vi "Main.vi"() -> ()   [LabVIEW 2012]
uses:
  MeasureDialogButton.ctl
  SourceDialogButton.ctl
  TriggerDialogButton.ctl
  DUTDisplayData.ctl
  DUTDialogButton.ctl
  LogDialogButton.ctl
  driver/Public/Controls/SMU.ctl
  DisplayDataGlobalAction.ctl
  UIActionQueueElement.ctl
  UIAction.ctl
  SetupGlobalAction.ctl
  HardwareActionQueueElement.ctl
  HardwareAction.ctl
  HardwareAbortGlobalAction.ctl
  LogActionQueueElement.ctl
  LogAction.ctl
  DisplayDataChartDialogGlobalAction.ctl
  driver/Keithley-2602.lvlib
  libs/LV-Utilities/LV-Utilities.lvlib
panel:
  in  "CREATE CHART":bool
  in  "Hardware START":bool
  out "Hardware Running?":bool
  in  "LOG START":bool
  out "Log Running?":bool
  out "Digital IO Port":bool[](array[boolean])
  out "Setup File":path
  in  "RESET":bool
  in  "SAVE":bool
  in  "OPEN":bool
  in  "SHOW LOG DIALOG":T1
  in  "SHOW DUT DIALOG":T2
  in  "SHOW SOURCE DIALOG":T3
  in  "SHOW TRIGGER DIALOG":T4
  in  "SHOW MEASURE DIALOG":T5
  out "System SMU B DUT Display Data":T6[](array[typedef]) {"Resistance (Ohm)" format="%_4p"; "Current (A)" format="%_4p"; "Voltage (V)" format="%_4p"}
  out "System SMU A DUT Display Data":T6[](array[typedef]) {"Resistance (Ohm)" format="%_4p"; "Current (A)" format="%_4p"; "Voltage (V)" format="%_4p"}
  out "Log File":path
  in  "DONE":bool
  # "RUN"
  # "LOG"
  # "DIGITAL IO"
  # "1"
  # "2"
  # "3"
  # "4"
  # "5"
  # "6"
  # "7"
  # "8"
  # "9"
  # "10"
  # "11"
  # "12"
  # "13"
  # "14"
  # "SETUP"
  # "SMU B"
  # "SMU A"
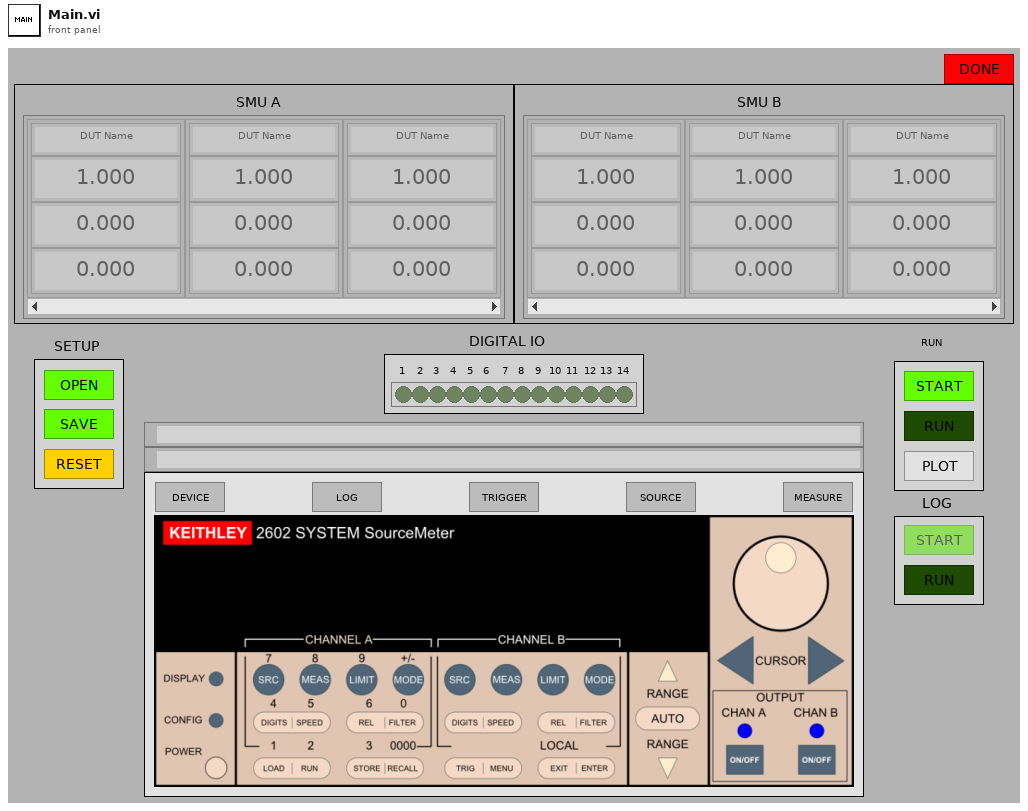
[diagram p1: front panel]
types:
  T1 = typedef "LogDialogButton.ctl" = bool
  T2 = typedef "DUTDialogButton.ctl" = bool
  T3 = typedef "SourceDialogButton.ctl" = bool
  T4 = typedef "TriggerDialogButton.ctl" = bool
  T5 = typedef "MeasureDialogButton.ctl" = bool
  T6 = typedef "DUTDisplayData.ctl" = cluster{"Name":string, "Voltage (V)":dbl, "Current (A)":dbl, "Resistance (Ohm)":dbl}
  T7 = typedef "ExecutableConfiguration.ctl" = cluster{"GPIB ID":u8, "GPIB Board":u8, "Default Data Folder":path, "Default Setup Folder":path}
  T8 = typedef "DataStructures.ctl" = cluster{"Display Data":refnum<notifier>, "Log Data":refnum<queue>}
  T9 = typedef "ActionQueues.ctl" = cluster{"UI Action":refnum<queue>, "Hardware Action":refnum<queue>, "Log Action":refnum<queue>}
  T10 = typedef "DisplayDataGlobalAction.ctl" = enum16{"Get", "Set"}
  T11 = typedef "Keithley-2602.lvlib/SMU.ctl" = enum16{"A", "B"}
  T12 = typedef "SetupGlobalAction.ctl" = enum16{"Get", "Set", "Reset"}
  T13 = enum8{"Enabled", "Disabled", "Disabled and Grayed Out"}
  T14 = typedef "UIActionQueueElement.ctl" = cluster{"Action":T15, "Data":variant}
  T15 = typedef "UIAction.ctl" = enum16{"Initialize", "Configure Trigger", "Configure Measure", "Configure Source", "Configure DUT", "Configure Log", "Configure Open", "Configure Save", "Configure Reset", "Hardware Start", "Hardware Started", "Hardware Stop", "Hardware Stopped", "Log Arm", "Log Start", "Log Started", "Log Stop", "Log Stopped", "Create Chart", "Error", "Shutdown"}
  T16 = typedef "HardwareActionQueueElement.ctl" = cluster{"Action":T17, "Data":variant}
  T17 = typedef "HardwareAction.ctl" = enum16{"Initialize", "Start", "Run", "Stop", "Error", "Shutdown"}
  T18 = typedef "HardwareAbortGlobalAction.ctl" = enum16{"Set", "Get"}
  T19 = typedef "LogActionQueueElement.ctl" = cluster{"Action":T20, "Data":variant}
  T20 = typedef "LogAction.ctl" = enum16{"Initialize", "Start", "Arm", "Create", "Write", "Close", "Rearm", "Stop", "Error", "Shutdown"}
  T21 = typedef "DisplayDataChartDialogGlobalAction.ctl" = enum16{"Create", "Close"}
  T22 = typedef "HardwareDisplayData.ctl" = cluster{"DUT Names":string[][], "SMU":dbl[][], "Port":bool[]}
  T23 = typedef "Setup.ctl" = cluster{"DUT":T24, "Log":T26, "Trigger":T34, "Sources":T40[], "Measures":T42[]}
  T24 = typedef "DUTConfiguration.ctl" = cluster{"Count":u32, "Wirings":T25[], "Names":string[][]}
  T25 = typedef "Keithley-2602.lvlib/SMUSense.ctl" = enum16{"Local (2-wire)", "Remote (4-wire)", "Calibration"}
  T26 = typedef "LogConfiguration.ctl" = cluster{"Start":T27, "Rollover":T30, "Stop":T32}
  T27 = typedef "LogStartConfiguration.ctl" = cluster{"Trigger Type":T28, "Timer (sec)":dbl, "Digital IO Line":u8, "Digital IO Edge":T29}
  T28 = typedef "LogStartTriggerType.ctl" = enum16{"Immediate", "User", "Timer", "Digital IO"}
  T29 = typedef "LogDigitalIOTriggerEdge.ctl" = enum16{"Rising", "Falling"}
  T30 = typedef "LogRolloverConfiguration.ctl" = cluster{"Trigger Type":T31, "Timer (sec)":dbl, "File Size (MB)":u32, "Digital IO Line":u8, "Digital IO Edge":T29}
  T31 = typedef "LogRolloverTriggerType.ctl" = enum16{"None", "Timer", "File Size", "Digital IO"}
  T32 = typedef "LogStopConfiguration.ctl" = cluster{"Trigger Type":T33, "Timer (sec)":dbl, "File Size (MB)":u32, "Digital IO Line":u8, "Digital IO Edge":T29}
  T33 = typedef "LogStopTriggerType.ctl" = enum16{"None", "User", "Timer", "File Size", "Digital IO"}
  T34 = typedef "TriggerConfiguration.ctl" = cluster{"Input":T35, "Output":T38}
  T35 = typedef "TriggerInputConfiguration.ctl" = cluster{"Type":T36, "Timeout (ms)":u32, "Delay (ms)":u32, "Digital IO Line (1-14)":u8, "Digital IO Mode":T37}
  T36 = typedef "TriggerInputType.ctl" = enum16{"None", "Digital IO", "Bus"}
  T37 = typedef "Keithley-2602.lvlib/TriggerMode.ctl" = enum16{"Falling", "Rising", "Either", "Synchronous"}
  T38 = typedef "TriggerOutputConfiguration.ctl" = cluster{"Type":T39, "Delay (ms)":u32, "Digital IO Line (1-14)":u8, "Digital IO Mode":T37, "Digital IO Pulse Width (sec)":dbl}
  T39 = typedef "TriggerOutputType.ctl" = enum16{"None", "Digital IO", "Bus"}
  T40 = typedef "SourceConfiguration.ctl" = cluster{"Enabled?":bool, "Function":T41, "Level (V or A)":dbl, "Autorange Enabled?":bool, "High Limit (V or A)":dbl, "Low Limit (V or A)":dbl}
  T41 = typedef "SourceFunction.ctl" = enum16{"Voltage", "Current"}
  T42 = typedef "MeasureConfiguration.ctl" = cluster{"Enabled?":bool, "Count":u8, "Interval (sec)":dbl, "Voltage Auto Range Enabled?":bool, "Voltage High Limit (V or A)":dbl, "Voltage Low Limit (V or A)":dbl, "Current Auto Range Enabled?":bool, "Current High Limit (V or A)":dbl, "Current Low Limit (V or A)":dbl}
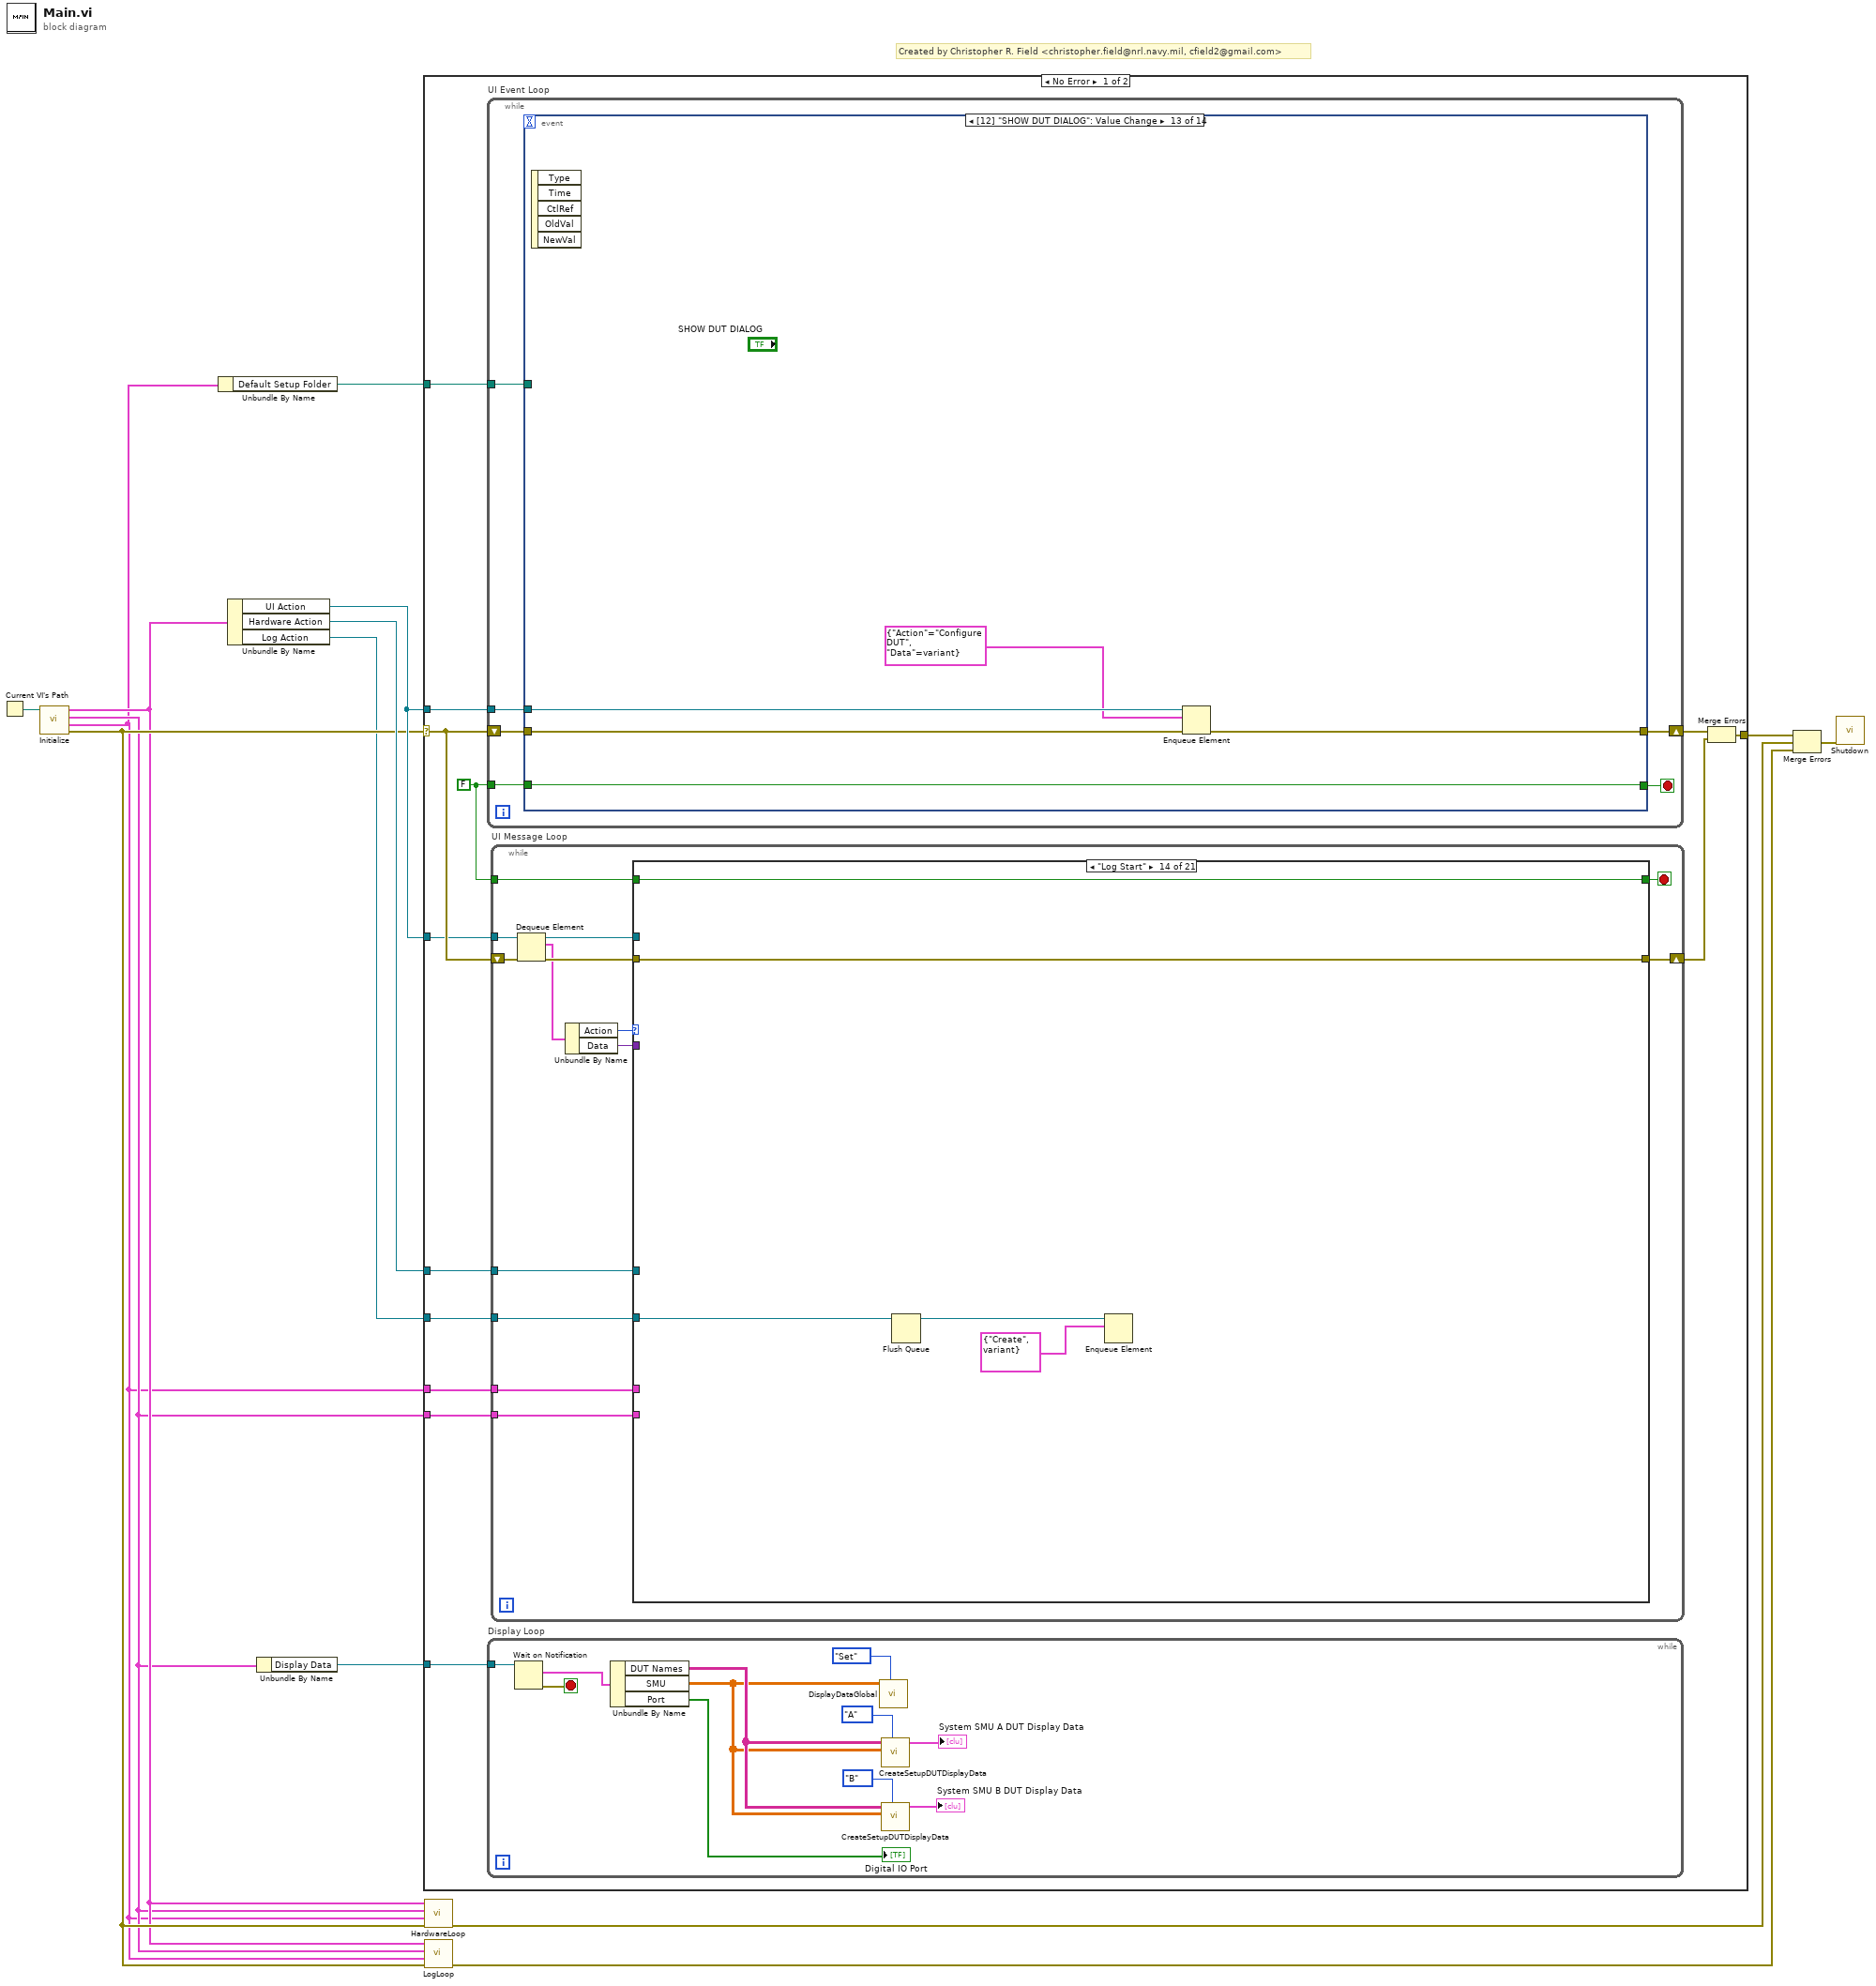
[diagram p0: block diagram]
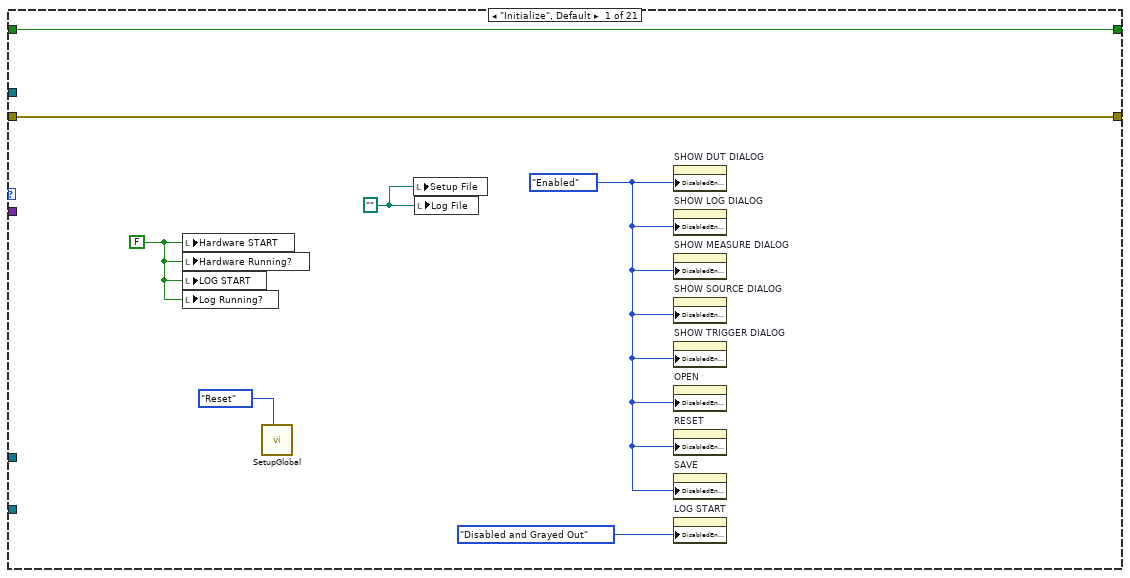
[diagram p2: hidden frame]
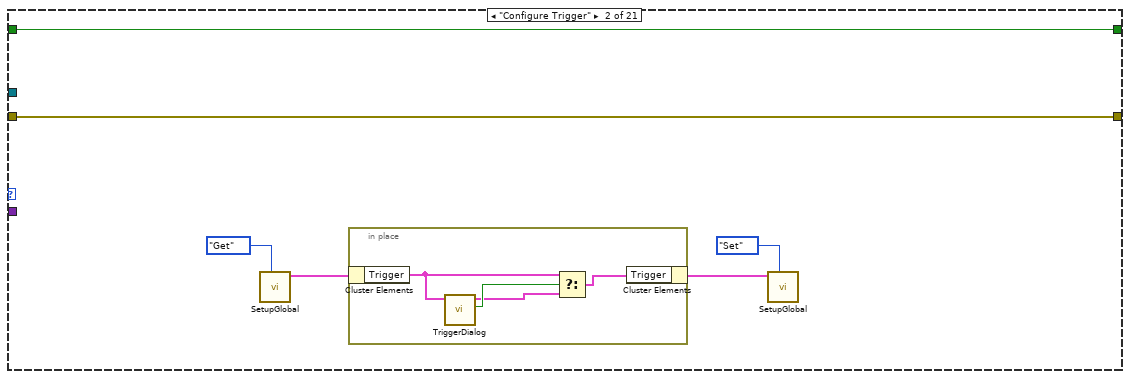
[diagram p3: hidden frame]
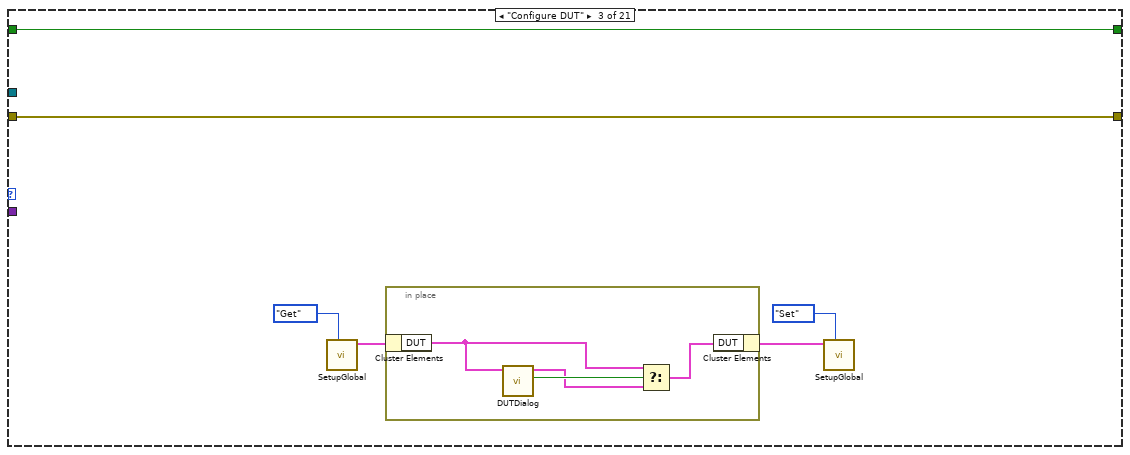
[diagram p4: hidden frame]
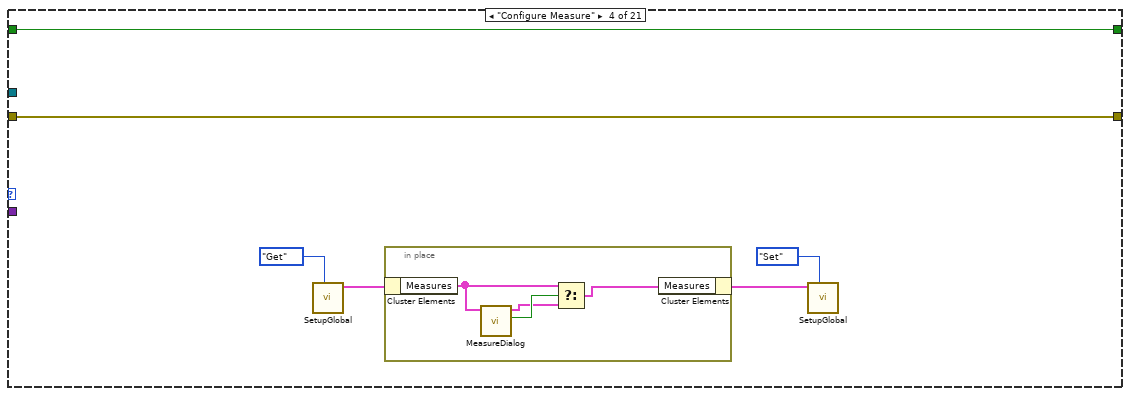
[diagram p5: hidden frame]
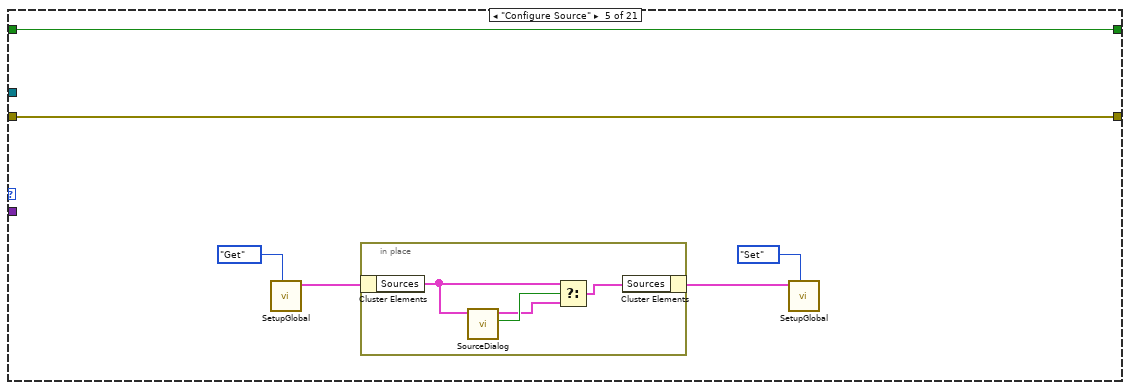
[diagram p6: hidden frame]
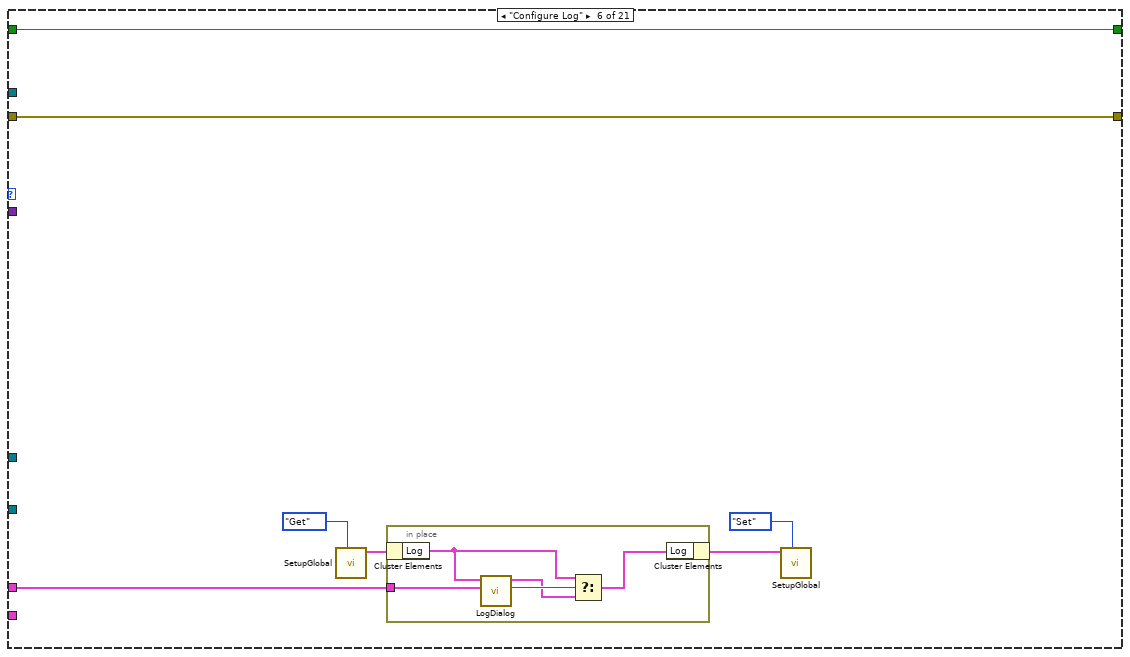
[diagram p7: hidden frame]
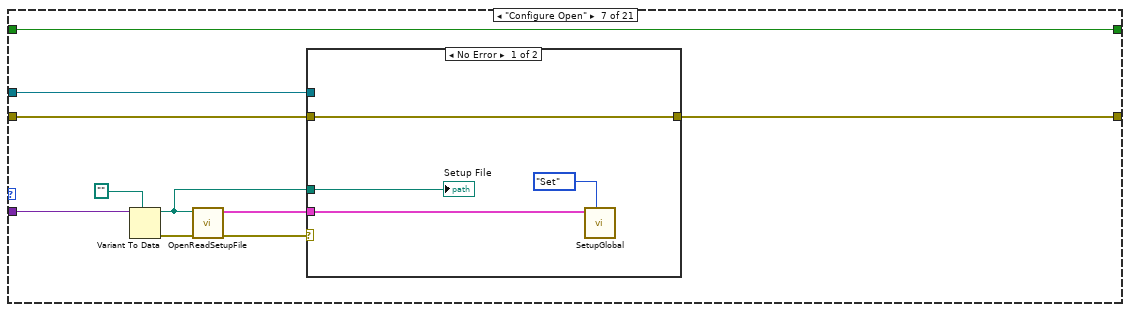
[diagram p8: hidden frame]
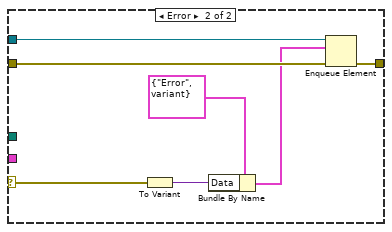
[diagram p9: hidden frame]
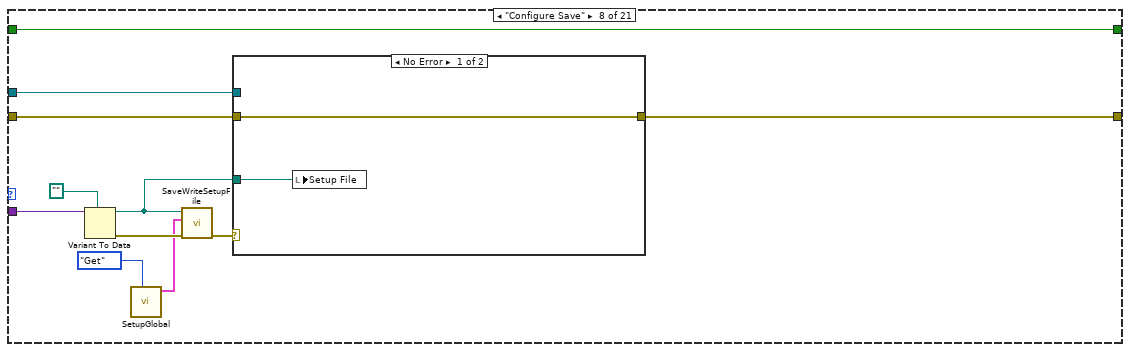
[diagram p10: hidden frame]
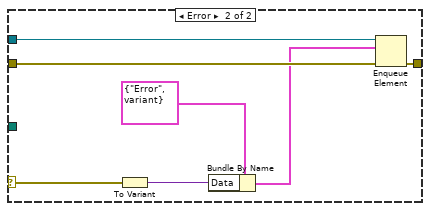
[diagram p11: hidden frame]
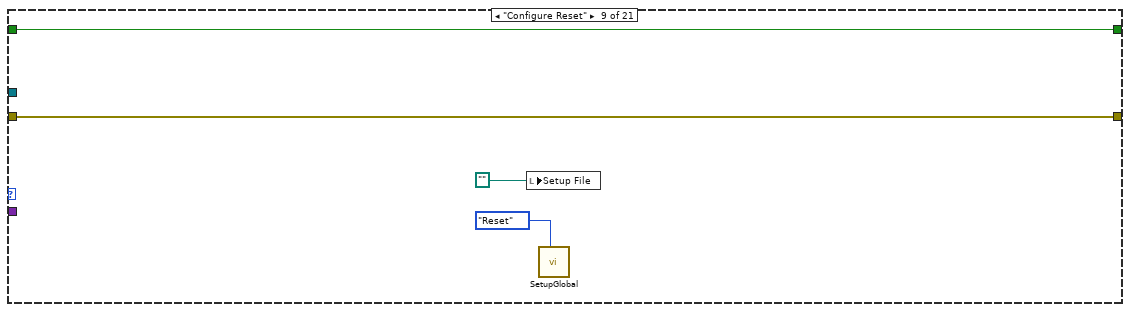
[diagram p12: hidden frame]
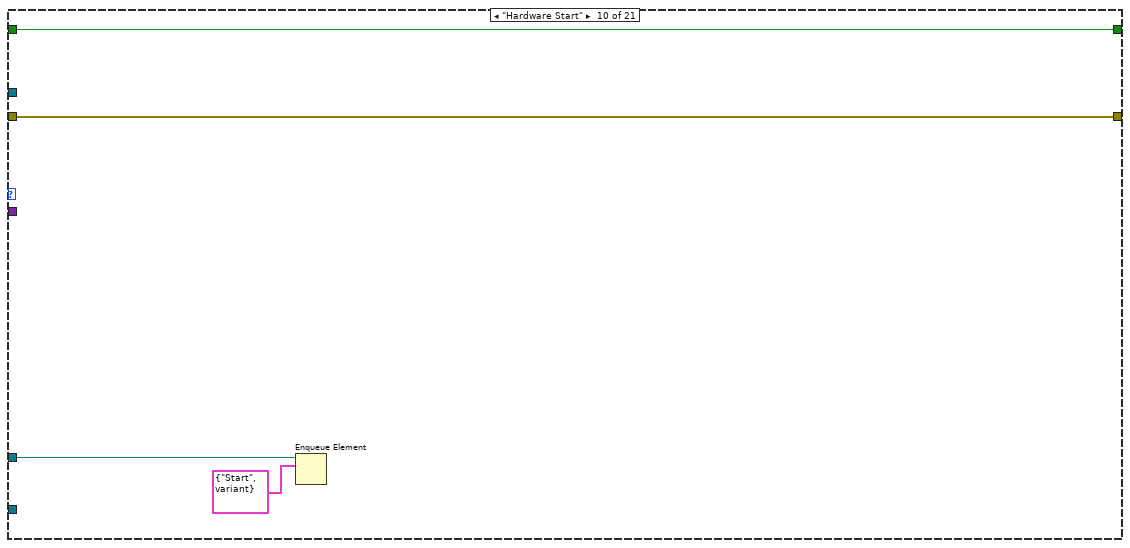
[diagram p13: hidden frame]
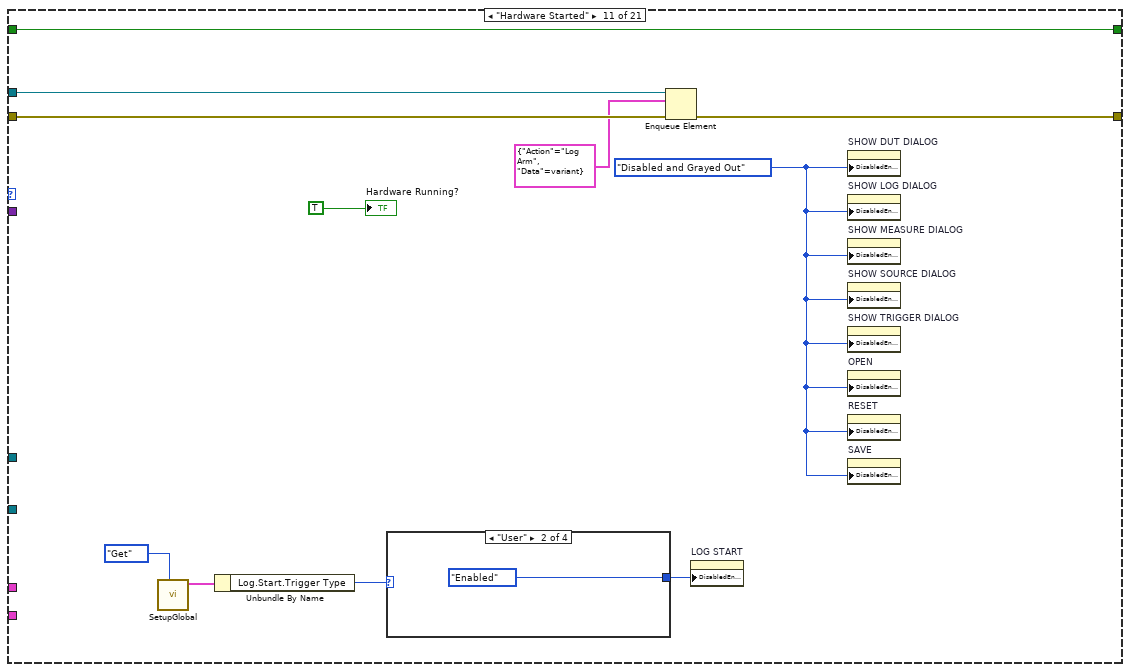
[diagram p14: hidden frame]
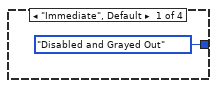
[diagram p15: hidden frame]
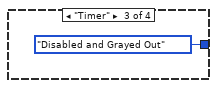
[diagram p16: hidden frame]
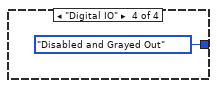
[diagram p17: hidden frame]
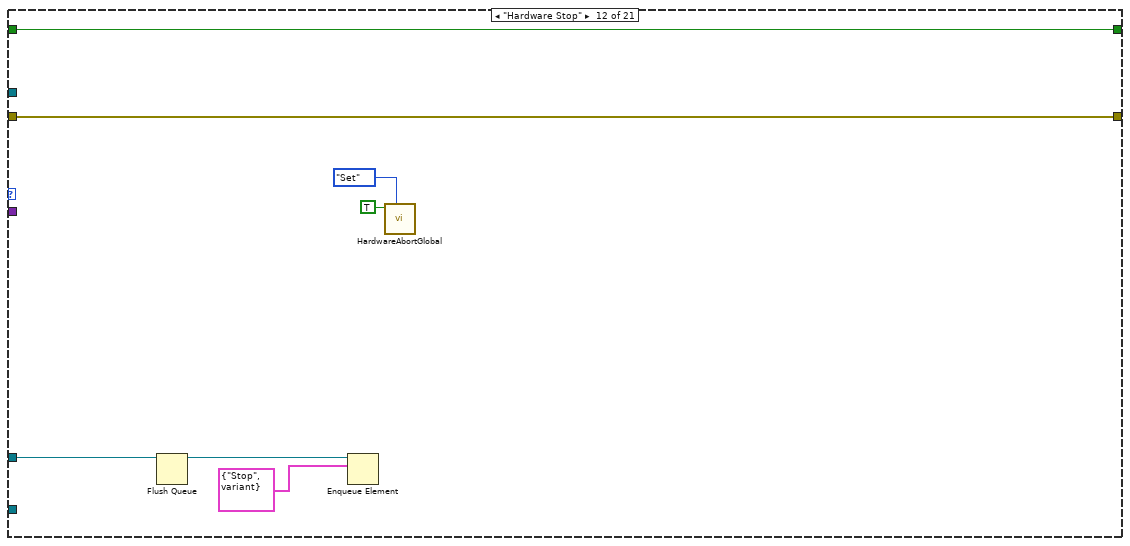
[diagram p18: hidden frame]
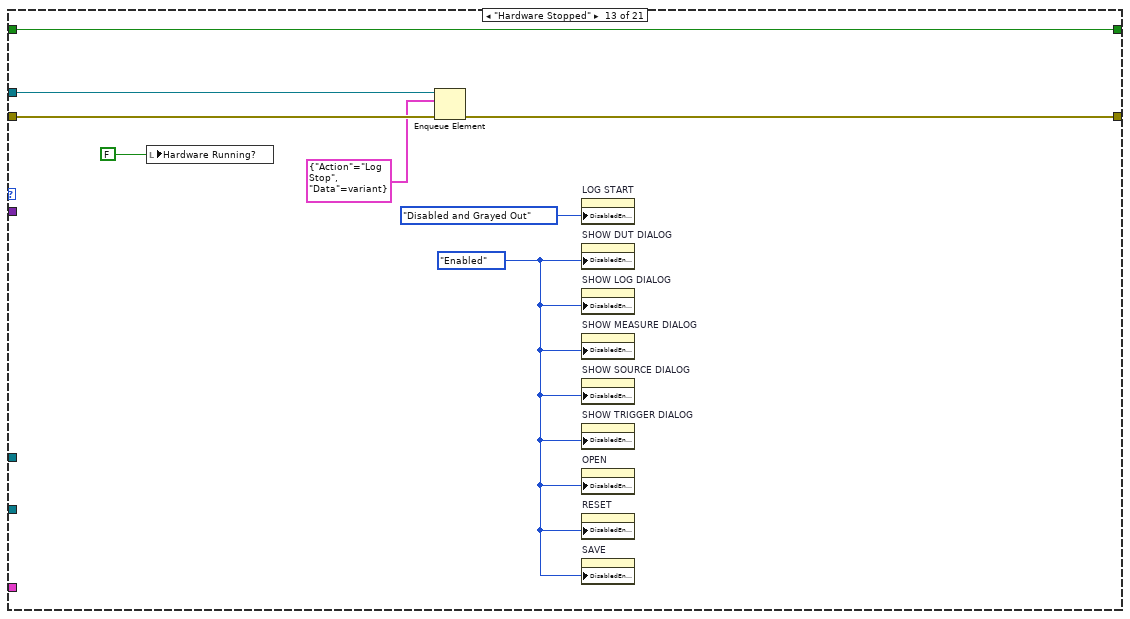
[diagram p19: hidden frame]
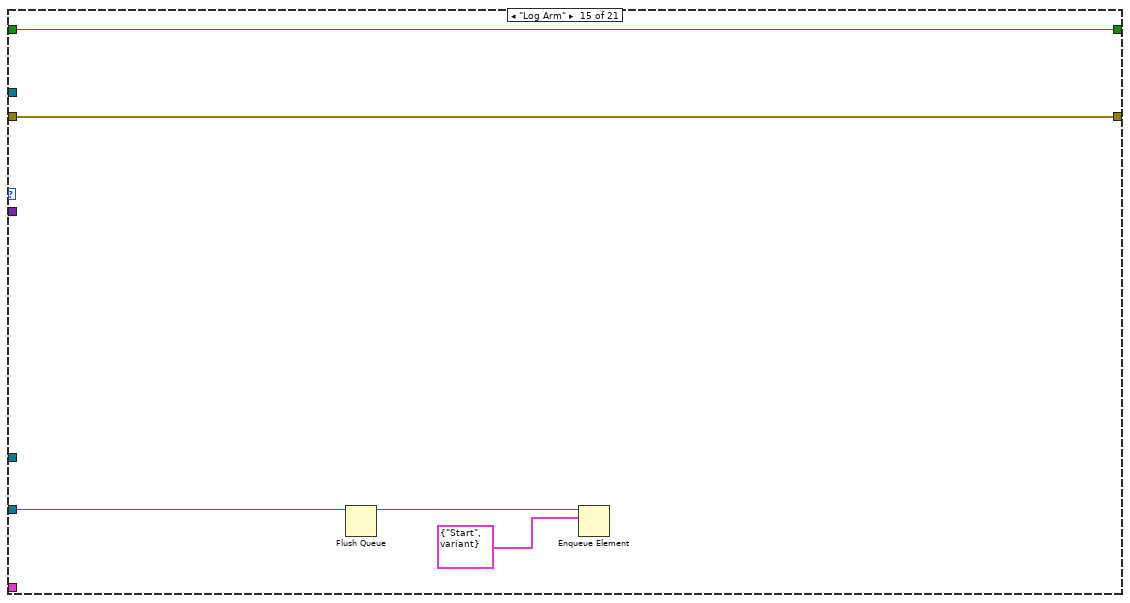
[diagram p20: hidden frame]
diagram:
  # "Created by Christopher R. Field <christopher.field@nrl.navy.mil, cfield2@gmail.com>"
  n1 = Current VI's Path() -> (path=w9:path)
  n2 = call "Initialize.vi"("VI Path"=w9) -> ("Error Out"=w7:errorcluster, "Executable Configuration"=w2:T7, "Data Structures"=w5:T8, "Action Queues"=w6:T9)  [unwired: 7 in]
  n3 = Unbundle By Name(w2) -> ("Default Setup Folder"=w1:path)
  n4 = Unbundle By Name(w6) -> ("UI Action"=w14:refnum<queue>, "Hardware Action"=w10:refnum<queue>, "Log Action"=w3:refnum<queue>)
  n5 = Unbundle By Name(w5) -> ("Display Data"=w8:refnum<notifier>)
  n6 = case shown="No Error" w7 {
    selector: w7 -> [w25 w373]
    tunnel: [w26 w373] -> w13
    tunnel: w14 -> [w22 _]
    tunnel: w14 -> [w21 _]
    tunnel: w10 -> [w20 _]
    tunnel: w8 -> [w19 _]
    tunnel: w5 -> [w18 _]
    tunnel: w2 -> [w17 _]
    tunnel: w3 -> [w16 _]
    tunnel: w1 -> [w15 _]
    frame No Error {
      w23 = FALSE
      n7 = while "UI Event Loop" {
        tunnel: w23 -> [w267]
        shift-right: [w264] -> w27
        shift-left: w25 -> [w265]
        tunnel: w21 -> [w263]
        tunnel: w15 -> [w262]
        stop <- w266 stop-if-true
        n8 = event shown="[12] \"SHOW DUT DIALOG\": Value Change" {
          selector: _ -> [_ _ _ _ _ _ _ _ _ _ _ _ _ _]
          dyn-events: _ -> [_ _ _ _ _ _ _ _ _ _ _ _ _ _]
          timeout: _ -> [_ _ _ _ _ _ _ _ _ _ _ _ _ _]
          tunnel: w267 -> [w269 w275 w280 w294 w310 w326 w331 w336 w338 w352 w357 w359 w367 w369]
          tunnel: [w269 w274 w280 w294 w310 w326 w331 w336 w338 w351 w357 w359 w367 w369] -> w266
          tunnel: w265 -> [w268 w271 w282 w285 w312 w324 w329 w334 w340 w347 w355 w361 w365 w371]
          tunnel: [w268 w272 w281 w286 w311 w323 w328 w333 w339 w350 w354 w360 w364 w370] -> w264
          tunnel: w263 -> [_ w273 w283 w287 w313 w325 w330 w335 w341 w348 w356 w362 w366 w372]
          tunnel: w262 -> [_ _ _ w284 w303 _ _ _ _ _ _ _ _ _]
          event Timeout {
            n9 = event-data() -> ()  [unwired: 1 in, 2 out]
          }
          event Panel Close? {
            n10 = event-data() -> ()  [unwired: 1 in, 3 out]
            n11 = Not(x=w275) -> (.not. x?=w274:bool)
            n12 = Enqueue Element(queue=w273, element=T14 {"Action"=enum."Shutdown", "Data"=variant}, error in (no error)=w271) -> (error out=w272:errorcluster)  [unwired: 1 in, 2 out]
            n13 = event-data("Discard?"=w274) -> ()  [unwired: 1 in, 1 out]
          }
          event "LOG START": Value Change {
            n14 = event-data() -> ()  [unwired: 1 in, 5 out]
            n15 = Select(t=T14 {"Action"=enum."Log Start", "Data"=variant} ("element"), s="LOG START", f=T14 {"Action"=enum."Log Stop", "Data"=variant} ("element")) -> (s? t:f=w276:T14)
            n16 = Enqueue Element(queue=w283, element=w276, error in (no error)=w282) -> (error out=w281:errorcluster)  [unwired: 1 in, 2 out]
          }
          event "OPEN": Value Change {
            n17 = event-data() -> ()  [unwired: 1 in, 5 out]
            n18 = call "SelectFile.vi"("Button Label"="Open", "Prompt"="Select Setup File", "File Description"="Setup File", "File Extension (.*)"=".xml", "Start Path"=w284) -> ("Cancelled?"=w289:bool, "Selected File Path"=w288:path)  [unwired: 4 in, 1 out]
            n19 = case shown="False" w289 {
              tunnel: w287 -> [w301 _]
              tunnel: w285 -> [w300 w302]
              tunnel: [w299 w302] -> w286
              tunnel: w288 -> [w296 _]
              frame False {
                n20 = To Variant(anything=w296) -> (Variant=w297:variant)
                n21 = Bundle By Name(cluster=T14 {"Action"=enum."Configure Open", "Data"=variant} ("element"), "Data"=w297) -> (w295:T14)
                n22 = Enqueue Element(queue=w301, element=w295, error in (no error)=w300) -> (error out=w299:errorcluster)  [unwired: 1 in, 2 out]
              }
              frame True {
              }
            }
          }
          event "SAVE": Value Change {
            n23 = event-data() -> ()  [unwired: 1 in, 5 out]
            n24 = call "SelectFile.vi"("Button Label"="Save", "Prompt"="Select Setup File", "File Description"="Setup File", "File Extension (.*)"=".xml", "Start Path"=w303) -> ("Cancelled?"=w305:bool, "Selected File Path"=w304:path)  [unwired: 4 in, 1 out]
            n25 = case shown="False" w305 {
              tunnel: w313 -> [w320 _]
              tunnel: w312 -> [w319 w321]
              tunnel: [w318 w321] -> w311
              tunnel: w304 -> [w315 _]
              frame False {
                n26 = To Variant(anything=w315) -> (Variant=w316:variant)
                n27 = Bundle By Name(cluster=T14 {"Action"=enum."Configure Save", "Data"=variant} ("element"), "Data"=w316) -> (w314:T14)
                n28 = Enqueue Element(queue=w320, element=w314, error in (no error)=w319) -> (error out=w318:errorcluster)  [unwired: 1 in, 2 out]
              }
              frame True {
              }
            }
          }
          event "RESET": Value Change {
            n29 = event-data() -> ()  [unwired: 1 in, 5 out]
            n30 = Enqueue Element(queue=w325, element=T14 {"Action"=enum."Configure Reset", "Data"=variant}, error in (no error)=w324) -> (error out=w323:errorcluster)  [unwired: 1 in, 2 out]
          }
          event Value Change {
            n31 = event-data() -> ()  [unwired: 1 in, 1 out]
            n32 = Enqueue Element(queue=w330, element=T14 {"Action"=enum."Configure Measure", "Data"=variant}, error in (no error)=w329) -> (error out=w328:errorcluster)  [unwired: 1 in, 2 out]
          }
          event Value Change {
            n33 = event-data() -> ()  [unwired: 1 in, 5 out]
            n34 = Enqueue Element(queue=w335, element=T14 {"Action"=enum."Configure Source", "Data"=variant}, error in (no error)=w334) -> (error out=w333:errorcluster)  [unwired: 1 in, 2 out]
          }
          event "Hardware START": Value Change {
            n35 = event-data() -> ()  [unwired: 1 in, 1 out]
            n36 = Select(t=T14 {"Action"=enum."Hardware Start", "Data"=variant} ("UI Action Queue Element"), s="Hardware START", f=T14 {"Action"=enum."Hardware Stop", "Data"=variant} ("UI Action Queue Element")) -> (s? t:f=w337:T14)
            n37 = Enqueue Element(queue=w341, element=w337, error in (no error)=w340) -> (error out=w339:errorcluster)  [unwired: 1 in, 2 out]
          }
          event "DONE": Value Change {
            n38 = event-data() -> ()  [unwired: 1 in, 5 out]
            n39 = Not(x=w352) -> (.not. x?=w351:bool)
            n40 = Flush Queue(queue=w348, error in (no error)=w347) -> (queue out=w345:refnum<queue>, error out=w346:errorcluster)  [unwired: 1 out]
            n41 = Enqueue Element(queue=w345, element=T14 {"Action"=enum."Shutdown", "Data"=variant}, error in (no error)=w346) -> (error out=w350:errorcluster)  [unwired: 1 in, 2 out]
          }
          event Value Change {
            n42 = event-data() -> ()  [unwired: 1 in, 5 out]
            n43 = Enqueue Element(queue=w356, element=T14 {"Action"=enum."Configure Trigger", "Data"=variant}, error in (no error)=w355) -> (error out=w354:errorcluster)  [unwired: 1 in, 2 out]
          }
          event "CREATE CHART": Value Change {
            n44 = event-data() -> ()  [unwired: 1 in, 5 out]
            n45 = Enqueue Element(queue=w362, element=T14 {"Action"=enum."Create Chart", "Data"=variant} ("UI Action Queue Element"), error in (no error)=w361) -> (error out=w360:errorcluster)  [unwired: 1 in, 2 out]
          }
          event Value Change {
            n46 = event-data() -> ()  [unwired: 1 in, 5 out]
            n47 = Enqueue Element(queue=w366, element=T14 {"Action"=enum."Configure DUT", "Data"=variant}, error in (no error)=w365) -> (error out=w364:errorcluster)  [unwired: 1 in, 2 out]
          }
          event Value Change {
            n48 = event-data() -> ()  [unwired: 1 in, 5 out]
            n49 = Enqueue Element(queue=w372, element=T14 {"Action"=enum."Configure Log", "Data"=variant}, error in (no error)=w371) -> (error out=w370:errorcluster)  [unwired: 1 in, 2 out]
          }
        }
      }
      n50 = while "Display Loop" {
        tunnel: w19 -> [w38]
        stop <- w37 stop-if-true
        n51 = Wait on Notification(notifier=w38) -> (notification=w36:T22, error out=w37:errorcluster)  [unwired: 3 in, 2 out]
        n52 = Unbundle By Name(w36) -> ("DUT Names"=w32:string[][], "SMU"=w29:dbl[][], "Port"=→"Digital IO Port":bool[])
        n53 = call "DisplayDataGlobal.vi"("Action"=DisplayDataGlobalAction."Set", "Set Value"=w29) -> ()  [unwired: 9 in, 1 out]
        n54 = call "CreateSetupDUTDisplayData.vi"("SMU"=SMU."A", "SMU Data"=w29, "DUT Names"=w32) -> ("DUT Display Data"=→"System SMU A DUT Display Data":T6[])  [unwired: 8 in]
        n55 = call "CreateSetupDUTDisplayData.vi"("SMU"=SMU."B", "SMU Data"=w29, "DUT Names"=w32) -> ("DUT Display Data"=→"System SMU B DUT Display Data":T6[])  [unwired: 8 in]
      }
      n56 = while "UI Message Loop" {
        shift-right: [w51] -> w24
        shift-left: w25 -> [w49]
        tunnel: w23 -> [w52]
        tunnel: w22 -> [w48]
        tunnel: w20 -> [w42]
        tunnel: w18 -> [w41]
        tunnel: w17 -> [w40]
        tunnel: w16 -> [w39]
        stop <- w50 stop-if-true
        n57 = Dequeue Element(queue=w48, error in (no error)=w49) -> (queue out=w46:refnum<queue>, element=w45:T14, error out=w47:errorcluster)  [unwired: 1 in, 1 out]
        n58 = Unbundle By Name(w45) -> ("Action"=w44:T15, "Data"=w43:variant)
        n59 = case shown="\"Log Start\"" w44 {
          tunnel: w52 -> [w59 w65 w75 w85 w95 w106 w121 w143 w156 w160 w171 w182 w190 w195 w200 w210 w221 w228 w239 w243 w257]
          tunnel: w47 -> [w58 w64 w74 w84 w94 w105 w113 w136 w155 w159 w167 w181 w187 w194 w197 w209 w220 w229 w238 w241 w254]
          tunnel: [w58 w64 w74 w84 w94 w105 w112 w135 w155 w159 w166 w181 w186 w194 w197 w209 w220 w229 w238 w241 w253] -> w51
          tunnel: [w59 w65 w75 w85 w95 w106 w121 w143 w156 w160 w171 w182 w190 w195 w200 w210 w221 w228 w239 w243 w256] -> w50
          tunnel: w46 -> [_ _ _ _ _ _ w114 w137 _ _ w168 _ w188 _ _ _ _ _ _ _ w255]
          tunnel: w43 -> [_ _ _ _ _ _ w120 w141 _ _ _ _ _ _ _ w208 _ _ _ w242 _]
          tunnel: w42 -> [_ _ _ _ _ _ _ _ _ w158 _ w179 _ _ _ _ _ _ _ _ w252]
          tunnel: w41 -> [_ _ _ _ _ _ _ _ _ _ _ _ _ _ _ _ _ _ _ _ _]
          tunnel: w40 -> [_ _ _ _ _ w104 _ _ _ _ _ _ _ _ _ _ _ _ _ _ _]
          tunnel: w39 -> [_ _ _ _ _ _ _ _ _ _ _ _ _ w193 w198 _ w219 _ _ _ w250]
          frame "Initialize", Default {
            w54 = T13."Enabled" ("Disabled")
            w55 = path ""
            w57 = FALSE ("START")
            n60 = local write "Hardware START"(w57) -> ()
            n61 = local write "Hardware Running?"(w57) -> ()
            n62 = local write "LOG START"(w57) -> ()
            n63 = local write "Log Running?"(w57) -> ()
            n64 = call "SetupGlobal.vi"("Action"=SetupGlobalAction."Reset") -> ()  [unwired: 10 in, 1 out]
            n65 = local write "Setup File"(w55) -> ()
            n66 = local write "Log File"(w55) -> ()
            n67 = property on="SHOW DUT DIALOG" class="Bool"("DisabledEnum"=w54) -> ()  [unwired: 2 in, 2 out]
            n68 = property on="SHOW LOG DIALOG" class="Bool"("DisabledEnum"=w54) -> ()  [unwired: 2 in, 2 out]
            n69 = property on="SHOW MEASURE DIALOG" class="Bool"("DisabledEnum"=w54) -> ()  [unwired: 2 in, 2 out]
            n70 = property on="SHOW SOURCE DIALOG" class="Bool"("DisabledEnum"=w54) -> ()  [unwired: 2 in, 2 out]
            n71 = property on="SHOW TRIGGER DIALOG" class="Bool"("DisabledEnum"=w54) -> ()  [unwired: 2 in, 2 out]
            n72 = property on="OPEN" class="Bool"("DisabledEnum"=w54) -> ()  [unwired: 2 in, 2 out]
            n73 = property on="RESET" class="Bool"("DisabledEnum"=w54) -> ()  [unwired: 2 in, 2 out]
            n74 = property on="SAVE" class="Bool"("DisabledEnum"=w54) -> ()  [unwired: 2 in, 2 out]
            n75 = property on="LOG START" class="Bool (strict)"("DisabledEnum"=T13."Disabled and Grayed Out" ("Disabled")) -> ()  [unwired: 2 in, 2 out]
          }
          frame "Configure Trigger" {
            n76 = call "SetupGlobal.vi"("Action"=SetupGlobalAction."Get") -> ("Value Out"=w62:T23)  [unwired: 10 in]
            n77 = in-place {
              n78 = in-place-cluster #1(w62) -> ("Trigger"=w66:T34)
              n79 = call "TriggerDialog.vi"("Trigger Configuration In"=w66) -> ("Cancelled"=w69:bool, "Trigger Configuration Out"=w68:T34)  [unwired: 8 in, 1 out]
              n80 = Select(t=w66, s=w69, f=w68) -> (s? t:f=w67:T34)
              n81 = in-place-cluster #1("Trigger"=w67) -> (w61:T23)
            }
            n82 = call "SetupGlobal.vi"("Action"=SetupGlobalAction."Set", "Set Value"=w61) -> ()  [unwired: 9 in, 1 out]
          }
          frame "Configure DUT" {
            n83 = call "SetupGlobal.vi"("Action"=SetupGlobalAction."Get") -> ("Value Out"=w72:T23)  [unwired: 10 in]
            n84 = in-place {
              n85 = in-place-cluster #2(w72) -> ("DUT"=w76:T24)
              n86 = call "DUTDialog.vi"("DUT Configuration In"=w76) -> ("Cancelled?"=w79:bool, "DUT Configuration Out"=w78:T24)  [unwired: 8 in, 1 out]
              n87 = Select(t=w76, s=w79, f=w78) -> (s? t:f=w77:T24)
              n88 = in-place-cluster #2("DUT"=w77) -> (w70:T23)
            }
            n89 = call "SetupGlobal.vi"("Action"=SetupGlobalAction."Set", "Set Value"=w70) -> ()  [unwired: 9 in, 1 out]
          }
          frame "Configure Measure" {
            n90 = call "SetupGlobal.vi"("Action"=SetupGlobalAction."Get") -> ("Value Out"=w82:T23)  [unwired: 10 in]
            n91 = in-place {
              n92 = in-place-cluster #3(w82) -> ("Measures"=w86:T42[])
              n93 = call "MeasureDialog.vi"("Measure Configuration In"=w86) -> ("Cancelled?"=w89:bool, "Measure Configuration Out"=w87:T42[])  [unwired: 8 in, 1 out]
              n94 = Select(t=w86, s=w89, f=w87) -> (s? t:f=w88:T42[])
              n95 = in-place-cluster #3("Measures"=w88) -> (w80:T23)
            }
            n96 = call "SetupGlobal.vi"("Action"=SetupGlobalAction."Set", "Set Value"=w80) -> ()  [unwired: 9 in, 1 out]
          }
          frame "Configure Source" {
            n97 = call "SetupGlobal.vi"("Action"=SetupGlobalAction."Get") -> ("Value Out"=w92:T23)  [unwired: 10 in]
            n98 = in-place {
              n99 = in-place-cluster #4(w92) -> ("Sources"=w96:T40[])
              n100 = call "SourceDialog.vi"("Source Configurations In"=w96) -> ("Cancelled?"=w99:bool, "Source Configurations Out"=w98:T40[])  [unwired: 8 in, 1 out]
              n101 = Select(t=w96, s=w99, f=w98) -> (s? t:f=w97:T40[])
              n102 = in-place-cluster #4("Sources"=w97) -> (w90:T23)
            }
            n103 = call "SetupGlobal.vi"("Action"=SetupGlobalAction."Set", "Set Value"=w90) -> ()  [unwired: 9 in, 1 out]
          }
          frame "Configure Log" {
            n104 = call "SetupGlobal.vi"("Action"=SetupGlobalAction."Get") -> ("Value Out"=w102:T23)  [unwired: 10 in]
            n105 = in-place {
              in-place-border: w104 -> [w108]
              n106 = in-place-cluster #5(w102) -> ("Log"=w107:T26)
              n107 = call "LogDialog.vi"("Executable Configuration"=w108, "Log Configuration In"=w107) -> ("Cancelled?"=w111:bool, "Log Configuration Out"=w110:T26)  [unwired: 7 in, 1 out]
              n108 = Select(t=w107, s=w111, f=w110) -> (s? t:f=w109:T26)
              n109 = in-place-cluster #5("Log"=w109) -> (w100:T23)
            }
            n110 = call "SetupGlobal.vi"("Action"=SetupGlobalAction."Set", "Set Value"=w100) -> ()  [unwired: 9 in, 1 out]
          }
          frame "Configure Open" {
            n111 = Variant To Data(type=path "", Variant=w120) -> (data=w115:path, error out=w118:errorcluster)  [unwired: 1 in]
            n112 = call "OpenReadSetupFile.vi"("Error In"=w118, "Setup File"=w115) -> ("Error Out"=w117:errorcluster, "Setup"=w116:T23)  [unwired: 8 in]
            n113 = case shown="No Error" w117 {
              selector: w117 -> [_ w127]
              tunnel: w116 -> [w122 _]
              tunnel: w115 -> [w125 _]
              tunnel: w114 -> [_ w132]
              tunnel: w113 -> [w124 w131]
              tunnel: [w124 w130] -> w112
              frame No Error {
                n114 = call "SetupGlobal.vi"("Action"=SetupGlobalAction."Set", "Set Value"=w122) -> ()  [unwired: 9 in, 1 out]
                "Setup File" <- w125
              }
              frame Error {
                n115 = To Variant(anything=w127) -> (Variant=w128:variant)
                n116 = Bundle By Name(cluster=T14 {"Action"=enum."Error", "Data"=variant} ("element"), "Data"=w128) -> (w126:T14)
                n117 = Enqueue Element(queue=w132, element=w126, error in (no error)=w131) -> (error out=w130:errorcluster)  [unwired: 1 in, 2 out]
              }
            }
          }
          frame "Configure Save" {
            n118 = Variant To Data(type=path "", Variant=w141) -> (data=w139:path, error out=w140:errorcluster)  [unwired: 1 in]
            n119 = call "SetupGlobal.vi"("Action"=SetupGlobalAction."Get") -> ("Value Out"=w133:T23)  [unwired: 10 in]
            n120 = call "SaveWriteSetupFile.vi"("Error In"=w140, "Setup"=w133, "Save File"=w139) -> ("Error Out"=w138:errorcluster)  [unwired: 8 in]
            n121 = case shown="No Error" w138 {
              selector: w138 -> [_ w147]
              tunnel: w139 -> [w145 _]
              tunnel: w137 -> [_ w152]
              tunnel: w136 -> [w144 w151]
              tunnel: [w144 w150] -> w135
              frame No Error {
                n122 = local write "Setup File"(w145) -> ()
              }
              frame Error {
                n123 = To Variant(anything=w147) -> (Variant=w148:variant)
                n124 = Bundle By Name(cluster=T14 {"Action"=enum."Error", "Data"=variant} ("element"), "Data"=w148) -> (w146:T14)
                n125 = Enqueue Element(queue=w152, element=w146, error in (no error)=w151) -> (error out=w150:errorcluster)  [unwired: 1 in, 2 out]
              }
            }
          }
          frame "Configure Reset" {
            n126 = local write "Setup File"(path "") -> ()
            n127 = call "SetupGlobal.vi"("Action"=SetupGlobalAction."Reset") -> ()  [unwired: 10 in, 1 out]
          }
          frame "Hardware Start" {
            n128 = Enqueue Element(queue=w158, element=T16 {"Action"=enum."Start", "Data"=variant} ("Hardware Action Queue Element")) -> ()  [unwired: 2 in, 3 out]
          }
          frame "Hardware Started" {
            w164 = T13."Disabled and Grayed Out" ("Disabled")
            n129 = call "SetupGlobal.vi"("Action"=SetupGlobalAction."Get") -> ("Value Out"=w162:T23)  [unwired: 10 in]
            n130 = Unbundle By Name(w162) -> ("Log.Start.Trigger Type"=w161:T28)
            n131 = case shown="\"User\"" w161 {
              tunnel: [T13."Disabled and Grayed Out" ("Disabled") T13."Enabled" ("Disabled") T13."Disabled and Grayed Out" ("Disabled") T13."Disabled and Grayed Out" ("Disabled")] -> w169
              frame "Immediate", Default {
              }
              frame "User" {
              }
              frame "Timer" {
              }
              frame "Digital IO" {
              }
            }
            n132 = Enqueue Element(queue=w168, element=T14 {"Action"=enum."Log Arm", "Data"=variant}, error in (no error)=w167) -> (error out=w166:errorcluster)  [unwired: 1 in, 2 out]
            n133 = property on="LOG START" class="Bool (strict)"("DisabledEnum"=w169) -> ()  [unwired: 2 in, 2 out]
            n134 = property on="SHOW DUT DIALOG" class="Bool"("DisabledEnum"=w164) -> ()  [unwired: 2 in, 2 out]
            n135 = property on="SHOW LOG DIALOG" class="Bool"("DisabledEnum"=w164) -> ()  [unwired: 2 in, 2 out]
            n136 = property on="SHOW MEASURE DIALOG" class="Bool"("DisabledEnum"=w164) -> ()  [unwired: 2 in, 2 out]
            n137 = property on="SHOW SOURCE DIALOG" class="Bool"("DisabledEnum"=w164) -> ()  [unwired: 2 in, 2 out]
            n138 = property on="SHOW TRIGGER DIALOG" class="Bool"("DisabledEnum"=w164) -> ()  [unwired: 2 in, 2 out]
            n139 = property on="OPEN" class="Bool"("DisabledEnum"=w164) -> ()  [unwired: 2 in, 2 out]
            n140 = property on="RESET" class="Bool"("DisabledEnum"=w164) -> ()  [unwired: 2 in, 2 out]
            n141 = property on="SAVE" class="Bool"("DisabledEnum"=w164) -> ()  [unwired: 2 in, 2 out]
            "Hardware Running?" <- TRUE ("Run Running?")
          }
          frame "Hardware Stop" {
            n142 = Flush Queue(queue=w179) -> (queue out=w178:refnum<queue>)  [unwired: 1 in, 2 out]
            n143 = Enqueue Element(queue=w178, element=T16 {"Action"=enum."Stop", "Data"=variant}) -> ()  [unwired: 2 in, 3 out]
            n144 = call "HardwareAbortGlobal.vi"("Action"=HardwareAbortGlobalAction."Set", "Set Value"=TRUE) -> ()  [unwired: 9 in, 1 out]
          }
          frame "Hardware Stopped" {
            w183 = T13."Enabled" ("Disabled")
            n145 = local write "Hardware Running?"(FALSE ("Hardware Armed?")) -> ()
            n146 = Enqueue Element(queue=w188, element=T14 {"Action"=enum."Log Stop", "Data"=variant}, error in (no error)=w187) -> (error out=w186:errorcluster)  [unwired: 1 in, 2 out]
            n147 = property on="LOG START" class="Bool (strict)"("DisabledEnum"=T13."Disabled and Grayed Out" ("Disabled")) -> ()  [unwired: 2 in, 2 out]
            n148 = property on="SHOW DUT DIALOG" class="Bool"("DisabledEnum"=w183) -> ()  [unwired: 2 in, 2 out]
            n149 = property on="SHOW LOG DIALOG" class="Bool"("DisabledEnum"=w183) -> ()  [unwired: 2 in, 2 out]
            n150 = property on="SHOW MEASURE DIALOG" class="Bool"("DisabledEnum"=w183) -> ()  [unwired: 2 in, 2 out]
            n151 = property on="SHOW SOURCE DIALOG" class="Bool"("DisabledEnum"=w183) -> ()  [unwired: 2 in, 2 out]
            n152 = property on="SHOW TRIGGER DIALOG" class="Bool"("DisabledEnum"=w183) -> ()  [unwired: 2 in, 2 out]
            n153 = property on="OPEN" class="Bool"("DisabledEnum"=w183) -> ()  [unwired: 2 in, 2 out]
            n154 = property on="RESET" class="Bool"("DisabledEnum"=w183) -> ()  [unwired: 2 in, 2 out]
            n155 = property on="SAVE" class="Bool"("DisabledEnum"=w183) -> ()  [unwired: 2 in, 2 out]
          }
          frame "Log Start" {
            n156 = Flush Queue(queue=w193) -> (queue out=w192:refnum<queue>)  [unwired: 1 in, 2 out]
            n157 = Enqueue Element(queue=w192, element=T19 {"Action"=enum."Create", "Data"=variant}) -> ()  [unwired: 2 in, 3 out]
          }
          frame "Log Arm" {
            n158 = Flush Queue(queue=w198) -> (queue out=w199:refnum<queue>)  [unwired: 1 in, 2 out]
            n159 = Enqueue Element(queue=w199, element=T19 {"Action"=enum."Start", "Data"=variant}) -> ()  [unwired: 2 in, 3 out]
          }
          frame "Log Started" {
            w204 = TRUE ("Log Running?")
            n160 = call "SetupGlobal.vi"("Action"=SetupGlobalAction."Get") -> ("Value Out"=w202:T23)  [unwired: 10 in]
            n161 = Variant To Data(type=path "", Variant=w208) -> (data=→"Log File":path)  [unwired: 1 in, 1 out]
            n162 = Unbundle By Name(w202) -> ("Log.Stop.Trigger Type"=w201:T33)
            n163 = case shown="\"Timer\"" w201 {
              tunnel: [T13."Disabled and Grayed Out" ("Disabled") T13."Enabled" ("Disabled") T13."Enabled" ("Disabled") T13."Enabled" ("Disabled") T13."Enabled" ("Disabled")] -> w205
              frame "None", Default {
              }
              frame "User" {
              }
              frame "Timer" {
              }
              frame "File Size" {
              }
              frame "Digital IO" {
              }
            }
            n164 = local write "LOG START"(w204) -> ()
            n165 = property on="LOG START" class="Bool (strict)"("DisabledEnum"=w205) -> ()  [unwired: 2 in, 2 out]
            "Log Running?" <- w204
          }
          frame "Log Stop" {
            n166 = Flush Queue(queue=w219) -> (queue out=w218:refnum<queue>, error out=w217:errorcluster)  [unwired: 1 in, 1 out]
            n167 = Enqueue Element(queue=w218, element=T19 {"Action"=enum."Stop", "Data"=variant}, error in (no error)=w217) -> ()  [unwired: 1 in, 3 out]
          }
          frame "Log Stopped" {
            w226 = FALSE ("Log Running?")
            n168 = call "SetupGlobal.vi"("Action"=SetupGlobalAction."Get") -> ("Value Out"=w224:T23)  [unwired: 10 in]
            n169 = Unbundle By Name(w224) -> ("Log.Start.Trigger Type"=w222:T28)
            n170 = case shown="\"User\"" w222 {
              tunnel: [T13."Disabled and Grayed Out" ("Disabled") w231 T13."Disabled and Grayed Out" ("Disabled") T13."Disabled and Grayed Out" ("Disabled")] -> w225
              frame "Immediate", Default {
              }
              frame "User" {
                n171 = local read "Hardware Running?"() -> (w234:bool)
                n172 = Select(t=T13."Enabled" ("Disabled"), s=w234, f=T13."Disabled and Grayed Out") -> (s? t:f=w231:T13)
              }
              frame "Timer" {
              }
              frame "Digital IO" {
              }
            }
            n173 = local write "Log Running?"(w226) -> ()
            n174 = local write "LOG START"(w226) -> ()
            n175 = local write "Log File"(path "") -> ()
            n176 = property on="LOG START" class="Bool (strict)"("DisabledEnum"=w225) -> ()  [unwired: 2 in, 2 out]
          }
          frame "Create Chart" {
            n177 = call "DisplayDataChartDialogGlobal.vi"("Action"=DisplayDataChartDialogGlobalAction."Create") -> ()  [unwired: 11 in]
          }
          frame "Error" {
            n178 = Variant To Data(type=w241, Variant=w242) -> (data=w240:errorcluster)  [unwired: 1 in, 1 out]
            n179 = call <vilib>:"General Error Handler.vi"("error in (no error)"=w240) -> ()  [unwired: 10 in, 5 out]
          }
          frame "Shutdown" {
            n180 = Release Queue(queue=w255, error in (no error)=w254) -> (error out=w253:errorcluster)  [unwired: 1 in, 2 out]
            n181 = Flush Queue(queue=w252) -> (queue out=w247:refnum<queue>)  [unwired: 1 in, 2 out]
            n182 = Flush Queue(queue=w250) -> (queue out=w249:refnum<queue>)  [unwired: 1 in, 2 out]
            n183 = Not(x=w257) -> (.not. x?=w256:bool)
            n184 = local read "Hardware START"() -> (w246:bool)
            n185 = Enqueue Element(queue=w249, element=T19 {"Action"=enum."Shutdown", "Data"=variant}) -> ()  [unwired: 2 in, 3 out]
            n186 = case shown="True" w246 {
              tunnel: w247 -> [w258 w260]
              tunnel: [w258 w259] -> w245
              frame False {
              }
              frame True {
                n187 = Enqueue Element(queue=w260, element=T16 {"Action"=enum."Stop", "Data"=variant}) -> (queue out=w259:refnum<queue>)  [unwired: 2 in, 2 out]
              }
            }
            n188 = call "DisplayDataChartDialogGlobal.vi"("Action"=DisplayDataChartDialogGlobalAction."Close") -> ()  [unwired: 11 in]
            n189 = Enqueue Element(queue=w245, element=T16 {"Action"=enum."Shutdown", "Data"=variant}) -> ()  [unwired: 2 in, 3 out]
          }
        }
      }
      n190 = Merge Errors(w27, w24) -> (w26:errorcluster)
    }
    frame Error {
    }
  }
  n191 = call "HardwareLoop.vi"("Error In"=w7, "Executable Configuration"=w2, "Data Structures"=w5, "Action Queues"=w6) -> ("Error Out"=w11:errorcluster)  [unwired: 7 in]
  n192 = call "LogLoop.vi"("Error In"=w7, "Executable Configuration"=w2, "Data Structures"=w5, "Action Queues"=w6) -> ("Error Out"=w4:errorcluster)  [unwired: 7 in]
  n193 = Merge Errors(w13, w11, w4) -> (w12:errorcluster)
  n194 = call "Shutdown.vi"("Error In"=w12) -> ()  [unwired: 10 in, 1 out]
